vi "PXI-Change AO Gains (gracefully) q.vi"(0 "Multipliers in":dbl[](array[numeric]), 5 "Gains":dbl[](array[numeric]), 11 "error in (no error)":errorcluster) -> (15 "error out":errorcluster)   [LabVIEW 2015]
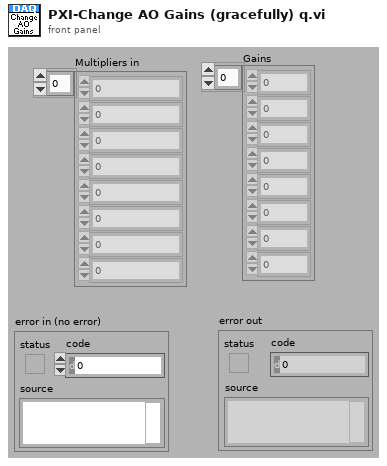
[diagram p1: front panel]
types:
  T1 = enum16{"Init", "Write", "Read", "Latch setup", "Compute comp."}
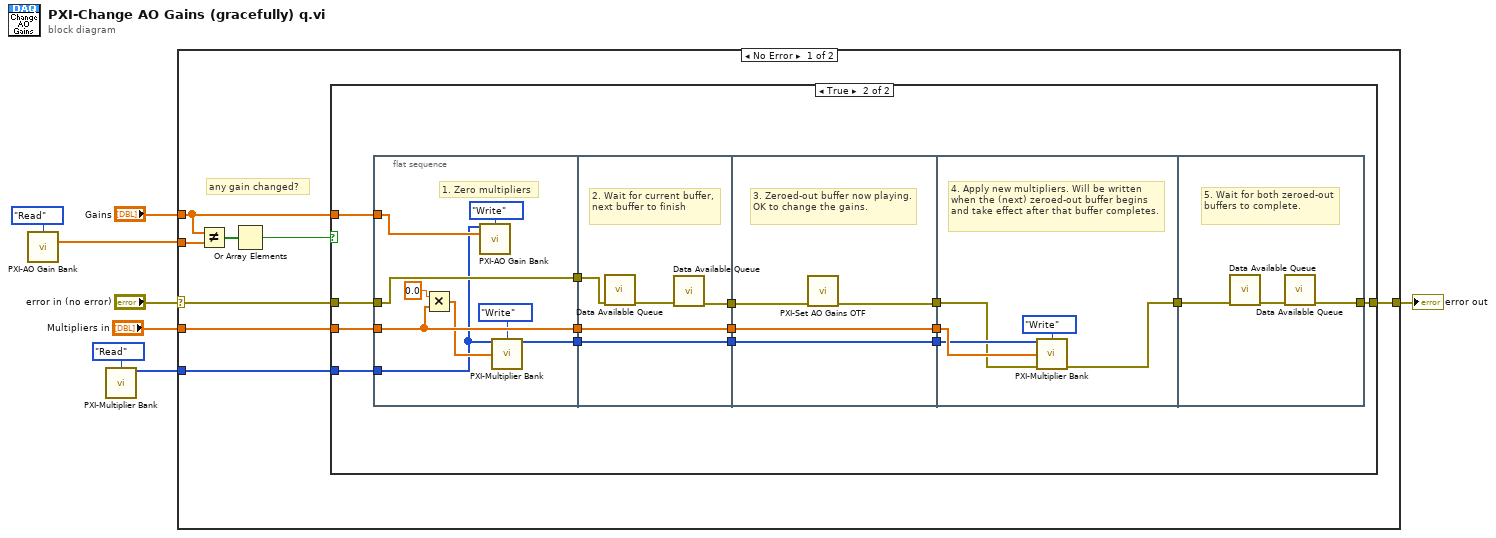
[diagram p0: block diagram]
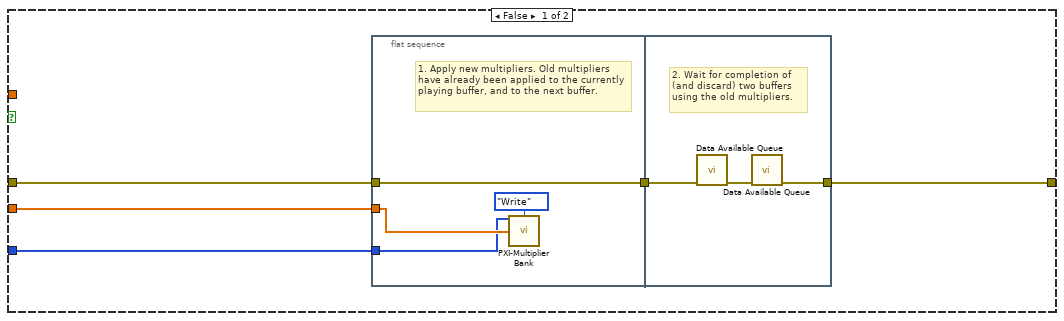
[diagram p2: hidden frame]
diagram:
  n1 = call "PXI-AO Gain Bank.vi"("Action"=T1."Read") -> ("Gains out"=w4:dbl[])  [unwired: 9 in, 5 out]
  n2 = call "PXI-Multiplier Bank.vi"("Action"=enum16{"Init", "Write", "Read"}."Read") -> ("Channels"=w1:i32[])  [unwired: 12 in, 2 out]
  n3 = case shown="No Error" "error in (no error)" {
    selector: "error in (no error)" -> [w10 w70]
    tunnel: w4 -> [w16 _]
    tunnel: [w14 w70] -> w8
    tunnel: "Multipliers in" -> [w13 _]
    tunnel: "Gains" -> [w12 _]
    tunnel: w1 -> [w9 _]
    frame No Error {
      # "any gain changed?"
      n4 = Not Equal?(x=w12, y=w16) -> (x != y?=w15:bool[])
      n5 = Or Array Elements(Boolean array=w15) -> (logical OR=w11:bool)
      n6 = case shown="True" w11 {
        tunnel: w10 -> [w19 w34]
        tunnel: [w18 w43] -> w14
        tunnel: w13 -> [w20 w42]
        tunnel: w12 -> [_ w36]
        tunnel: w9 -> [w17 w33]
        frame False {
          n7 = flat-sequence {
            tunnel: [w25] -> w21
            tunnel: w20 -> [w23]
            tunnel: w19 -> [w25]
            tunnel: w17 -> [w22]
            tunnel: [w26] -> w18
            tunnel: w21 -> [w28]
            frame #0 {
              # "1. Apply new multipliers. Old multipliers have already been applied to the currently playing buffer, and to the next buffer."
              n8 = call "PXI-Multiplier Bank.vi"("AO Channels"=w22, "Action"=enum16{"Init", "Write", "Read"}."Write", "Multipliers"=w23) -> ()  [unwired: 10 in, 3 out]
            }
            frame #1 {
              # "2. Wait for completion of (and discard) two buffers using the old multipliers."
              n9 = call "Data Available Queue.vi"("error in (no error)"=w28) -> ("error out"=w27:errorcluster)  [unwired: 11 in, 3 out]
              n10 = call "Data Available Queue.vi"("error in (no error)"=w27) -> ("error out"=w26:errorcluster)  [unwired: 11 in, 3 out]
            }
          }
        }
        frame True {
          n11 = flat-sequence {
            tunnel: w42 -> [w48]
            tunnel: [w48] -> w40
            tunnel: w36 -> [w50]
            tunnel: [w51] -> w35
            tunnel: w34 -> [w51]
            tunnel: w33 -> [w44]
            tunnel: [w46] -> w30
            tunnel: [w57] -> w41
            tunnel: w40 -> [w57]
            tunnel: [w55] -> w37
            tunnel: w35 -> [w54]
            tunnel: [w53] -> w31
            tunnel: w30 -> [w53]
            tunnel: [w60] -> w39
            tunnel: [w59] -> w38
            tunnel: w37 -> [w61]
            tunnel: w41 -> [w59]
            tunnel: [w58] -> w32
            tunnel: w31 -> [w58]
            tunnel: w39 -> [w63]
            tunnel: w38 -> [w65]
            tunnel: w32 -> [w64]
            tunnel: [w62] -> w29
            tunnel: [w67] -> w43
            tunnel: w29 -> [w69]
            frame #0 {
              # "1. Zero multipliers"
              n12 = Multiply(x=0.0 ("Slide 2"), y=w48) -> (x*y=w45:dbl[])
              n13 = call "PXI-AO Gain Bank.vi"("AO Channels"=w44, "Action"=T1."Write", "Gains"=w50) -> ()  [unwired: 7 in, 6 out]
              n14 = call "PXI-Multiplier Bank.vi"("AO Channels"=w44, "Action"=enum16{"Init", "Write", "Read"}."Write", "Multipliers"=w45) -> ("Channels"=w46:i32[])  [unwired: 10 in, 2 out]
            }
            frame #1 {
              # "2. Wait for current buffer, next buffer to finish"
              n15 = call "Data Available Queue.vi"("error in (no error)"=w54) -> ("error out"=w56:errorcluster)  [unwired: 11 in, 3 out]
              n16 = call "Data Available Queue.vi"("error in (no error)"=w56) -> ("error out"=w55:errorcluster)  [unwired: 11 in, 3 out]
            }
            frame #2 {
              # "3. Zeroed-out buffer now playing. OK to change the gains."
              n17 = call "PXI-Set AO Gains OTF.vi"("error in (no error)"=w61) -> ("error out"=w60:errorcluster)  [unwired: 10 in]
            }
            frame #3 {
              # "4. Apply new multipliers. Will be written when the (next) zeroed-out buffer begins and take effect after that buffer completes."
              n18 = call "PXI-Multiplier Bank.vi"("AO Channels"=w64, "Action"=enum16{"Init", "Write", "Read"}."Write", "Multipliers"=w65, "error in (no error)"=w63) -> ("error out"=w62:errorcluster)  [unwired: 9 in, 2 out]
            }
            frame #4 {
              # "5. Wait for both zeroed-out buffers to complete."
              n19 = call "Data Available Queue.vi"("error in (no error)"=w69) -> ("error out"=w68:errorcluster)  [unwired: 11 in, 3 out]
              n20 = call "Data Available Queue.vi"("error in (no error)"=w68) -> ("error out"=w67:errorcluster)  [unwired: 11 in, 3 out]
            }
          }
        }
      }
    }
    frame Error {
    }
  }
  "error out" <- w8
